vi "Meas Gen Sequence.vi"(8 "error in":errorcluster, 10 "DC bias compensate (False)":bool, 11 "sweep setup":T2 {"f list"."bias" format="%#_3p"; "f list"."level" format="%#_3p"; "f list"."fs [Hz]" format="%#_5p"; "f list"."time [s]" format="%#_3p"; "f list"."f/fs" format="%#_3p"; "f list"."periods" format="%#_3f"; "f list"."f [Hz]" format="%#_5p"}) -> (0 "error out":errorcluster, 3 "sequence":T1[](array[typedef]))   [LabVIEW 2013]
doc: "Generates measurement sequence (sweep/readings)."
uses:
  Meas Sweep Config.ctl
  Meas Freq Info.ctl
  meas_swp_mode.ctl
  meas_sweep_flist_mode.ctl
  Meas Sequence Item.ctl
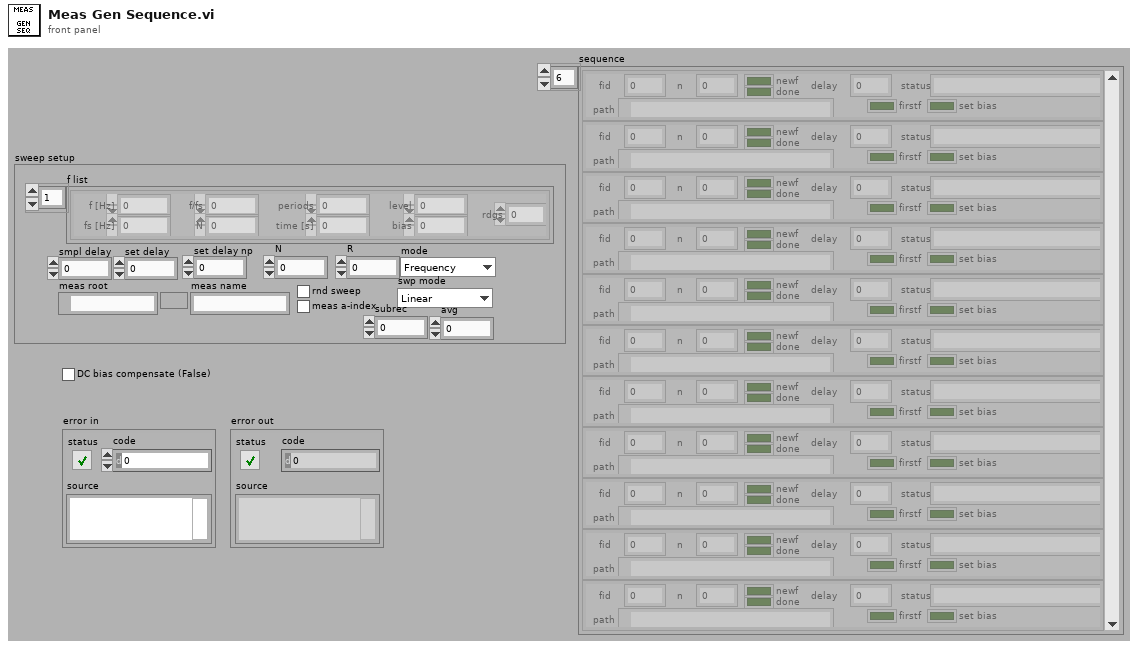
[diagram p1: front panel]
types:
  T1 = typedef "Meas Sequence Item.ctl" = cluster{"fid":i32, "n":i32, "newf":bool, "done":bool, "delay":dbl, "status":string, "path":path, "firstf":bool, "set bias":bool}
  T2 = typedef "Meas Sweep Config.ctl" = cluster{"N":i32, "R":i32, "f list":T3[], "smpl delay":dbl, "set delay":dbl, "set delay np":dbl, "meas root":path, "meas name":string, "meas a-index":bool, "rnd sweep":bool, "mode":T4, "swp mode":T5, "avg":i32, "subrec":i32}
  T3 = typedef "Meas Freq Info.ctl" = cluster{"f [Hz]":dbl, "periods":dbl, "f/fs":dbl, "time [s]":dbl, "fs [Hz]":dbl, "N":i32, "level":dbl, "bias":dbl, "rdgs":i32}
  T4 = typedef "meas_swp_mode.ctl" = enum16{"Frequency", "Level", "Bias"}
  T5 = typedef "meas_sweep_flist_mode.ctl" = enum16{"Linear", "Log10"}
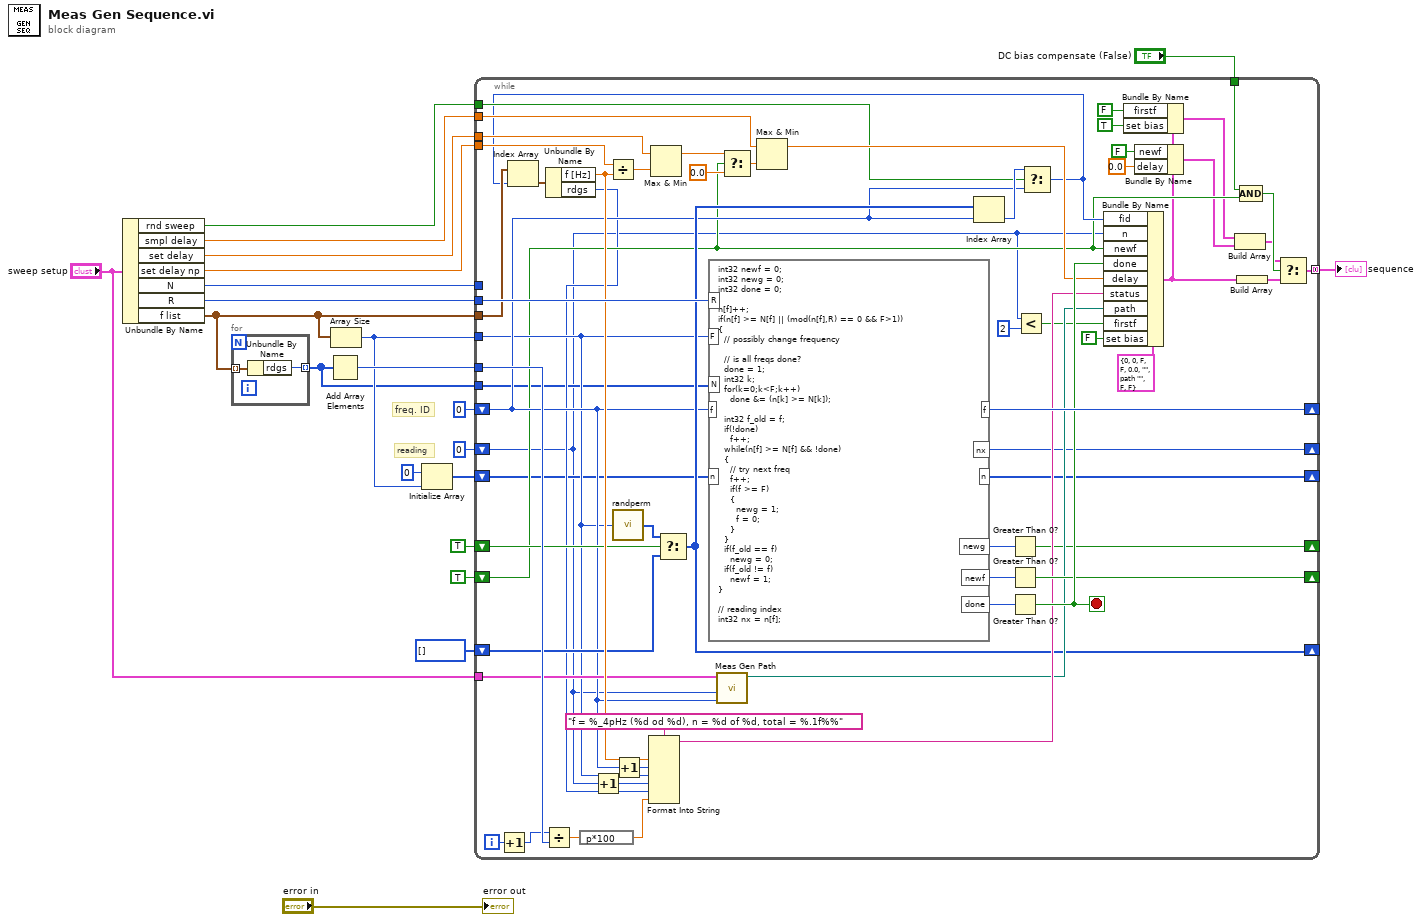
[diagram p0: block diagram]
diagram:
  # "reading"
  # "freq. ID"
  n1 = Unbundle By Name("sweep setup") -> ("rnd sweep"=w11:bool, "smpl delay"=w15:dbl, "set delay"=w16:dbl, "set delay np"=w17:dbl, "N"=w9:i32, "R"=w21:i32, "f list"=w7:T3[])
  n2 = for {
    tunnel: w7 -> [w23] mode=indexing
    tunnel: [w22] -> w1 mode=indexing
    n3 = Unbundle By Name(w23) -> ("rdgs"=w22:i32)
  }
  n4 = Add Array Elements(numeric array=w1) -> (sum=w6:i32)
  n5 = Array Size(array=w7) -> (size(s)=w4:i32)
  n6 = Initialize Array(0, w4) -> (w2:i32[])
  n7 = while {
    tunnel: w9 -> [_]
    tunnel: w21 -> [w85]
    tunnel: w4 -> [w47]
    shift-right: [w84] -> _
    shift-left: 0 -> [w49]
    shift-right: [w25] -> _
    shift-left: 0 -> [w24]
    tunnel: [w39] -> w19 mode=concatenating
    shift-right: [w79] -> _
    shift-left: TRUE -> [w42]
    tunnel: w7 -> [w78]
    tunnel: w17 -> [w76]
    tunnel: w16 -> [w74]
    tunnel: w15 -> [w70]
    tunnel: w6 -> [w60]
    tunnel: "sweep setup" -> [w58]
    shift-right: [w55] -> _
    shift-left: TRUE -> [w54]
    shift-right: [w51] -> _
    shift-left: i32[] [] -> [w52]
    tunnel: w11 -> [w48]
    tunnel: "DC bias compensate (False)" -> [w41]
    shift-right: [w27] -> _
    shift-left: w2 -> [w28]
    tunnel: w1 -> [w26]
    i -> [w64]
    stop <- w80 stop-if-true
    n8 = Increment(x=w64) -> (x+1=w59:i32)
    n9 = Divide(x=w59, y=w60) -> (x/y=w63:dbl)
    n10 = expression code="p*100"(w63) -> (w62:dbl)
    n11 = Increment(x=w24) -> (x+1=w65:i32)
    n12 = call "randperm.vi"("N"=w47) -> ("permutations"=w53:i32[])
    n13 = Increment(x=w49) -> (x+1=w66:i32)
    n14 = Select(t=w53, s=w54, f=w52) -> (s? t:f=w51:i32[])
    n15 = formula code="int32 newf = 0;\nint32 newg = 0;\nint32 done = 0;\n\nn[f]++;\nif(n[f] >= N[f] || (mod(n[f],R) == 0 && F>1))\n{\n  // possibly change frequency\n\n  // is all freqs done?\n  done = 1;\n  int32 k;\n  for(k=0;k<F;k++)\n    done &= (n[k] >= N[k]);\n  \n  int32 f_old = f;\n  if(!done)\n    f++;\n  while(n[f] >= N[f] && !done)\n  {\n    // try next freq\n    f++;\n    if(f >= F)\n    {\n      newg = 1;\n      f = 0;\n    }\n  }\n  if(f_old == f)\n    newg = 0;\n  if(f_old != f)\n    newf = 1;\n}\n\n// reading index\nint32 nx = n[f];"("F"=w47, "R"=w85, "f"=w49, "n"=w28, "N"=w26) -> ("f"=w84:i32, "nx"=w25:i32, "done"=w83:i32, "newf"=w82:i32, "newg"=w56:i32, "n"=w27:i32[])
    n16 = call "Meas Gen Path.vi"("f id"=w49, "n id"=w24, "swp cfg"=w58) -> ("meas path"=w57:path)  [unwired: 8 in]
    n17 = Index Array(array=w51, index=w49) -> (element=w50:i32)
    n18 = Greater Than 0?(x=w56) -> (x > 0?=w55:bool)
    n19 = Greater Than 0?(x=w82) -> (x > 0?=w79:bool)
    n20 = Greater Than 0?(x=w83) -> (x > 0?=w80:bool)
    n21 = Less?(x=w24, y=2 ("x")) -> (x < y?=w45:bool)
    n22 = Select(t=w50, s=w48, f=w49) -> (s? t:f=w46:i32)
    n23 = Index Array(array=w78, index=w46) -> (element=w77:T3)
    n24 = Unbundle By Name(w77) -> ("f [Hz]"=w67:dbl, "rdgs"=w29:i32)
    n25 = Divide(x=w76, y=w67) -> (x/y=w75:dbl)
    n26 = Format Into String(format string="f = %_4pHz (%d od %d), n = %d of %d, total = %.1f%%", w67, w66, w47, w65, w29, w62) -> (resulting string=w61:string)  [unwired: 2 in, 1 out]
    n27 = Max & Min(x=w74, y=w75) -> (max(x,y)=w73:dbl)  [unwired: 1 out]
    n28 = Select(t=w73, s=w42, f=0.0) -> (s? t:f=w71:dbl)
    n29 = Max & Min(x=w70, y=w71) -> (max(x,y)=w69:dbl)  [unwired: 1 out]
    n30 = Bundle By Name(cluster=T1 {"fid"=0, "n"=0, "newf"=FALSE, "done"=FALSE, "delay"=0.0, "status"="", "path"=path "", "firstf"=FALSE, "set bias"=FALSE} ("seq item"), "fid"=w46, "n"=w24, "newf"=w42, "done"=w80, "delay"=w69, "status"=w61, "path"=w57, "firstf"=w45, "set bias"=FALSE ("save rdg")) -> (w35:T1)
    n31 = Bundle By Name(cluster=w35, "firstf"=FALSE, "set bias"=TRUE ("save rdg")) -> (w40:T1)
    n32 = Bundle By Name(cluster=w35, "newf"=FALSE, "delay"=0.0) -> (w34:T1)
    n33 = Build Array(w40, w34) -> (w37:T1[])
    n34 = Build Array(w35) -> (w36:T1[])
    n35 = Compound Arithmetic op=AND(w41, w42) -> (w38:bool)
    n36 = Select(t=w37, s=w38, f=w36) -> (s? t:f=w39:T1[])
  }
  "sequence" <- w19
  "error out" <- "error in"
